vi "DHE_DRV_clear_table.vi"(11 "error in (no error)":errorcluster) -> (15 "error out":errorcluster)   [LabVIEW 2016]
doc: "This VI turns instrument power on (Flag=1) or off (Flag=0)."
uses:
  c/lib/libarcDHE.so
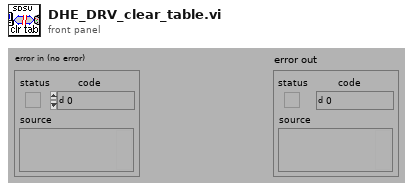
[diagram p1: front panel]
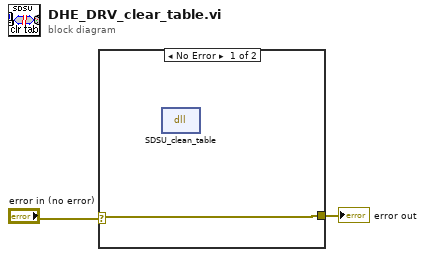
[diagram p0: block diagram]
diagram:
  n1 = case shown="No Error" "error in (no error)" {
    selector: "error in (no error)" -> [w3 w4]
    tunnel: [w3 w4] -> w2
    frame No Error {
      n2 = dll-call lib="home/simager/panview/PAN/Modules/SDSU/private/c/lib/libarcDHE.so" fn="SDSU_clean_table" label="clear_array"() -> ()  [unwired: 3 in, 3 out]
    }
    frame Error {
    }
  }
  "error out" <- w2
